vi "XS Electrode Write To Buffer.vi"(0 "XS Electrode Grid Array":bool[][](array[boolean])=[[FALSE, FALSE, FALSE], [FALSE, FALSE, FALSE], [FALSE, FALSE, FALSE], [FALSE, FALSE, FALSE], [FALSE, FALSE, FALSE], [FALSE, FALSE, FALSE]], 1 "64-bitmask Input":u64 format="%064b") -> (5 "64-bitmask Output":u64 format="%064b")   [LabVIEW 2017]
doc: "This VI will map the XS electrode grid array to ON-OFF bits in tehe 64 bit data buffer.\n\nAn array constant in this VI maps the XS electrode grid positions to the required HV channels."
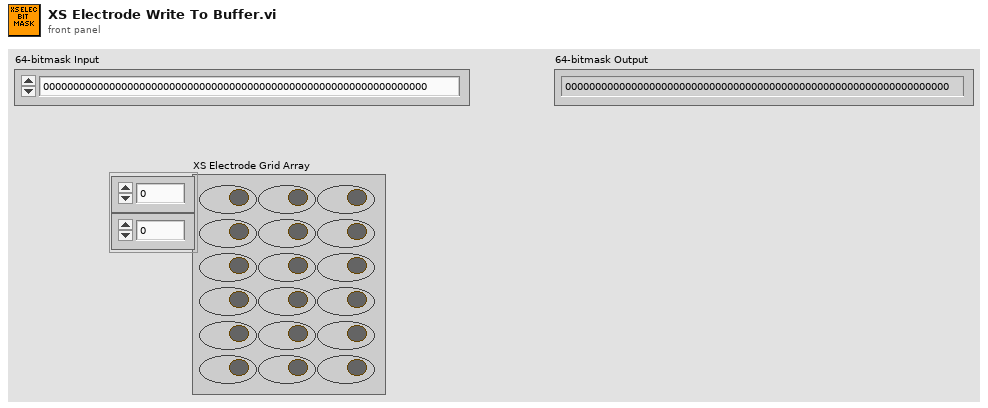
[diagram p1: front panel]
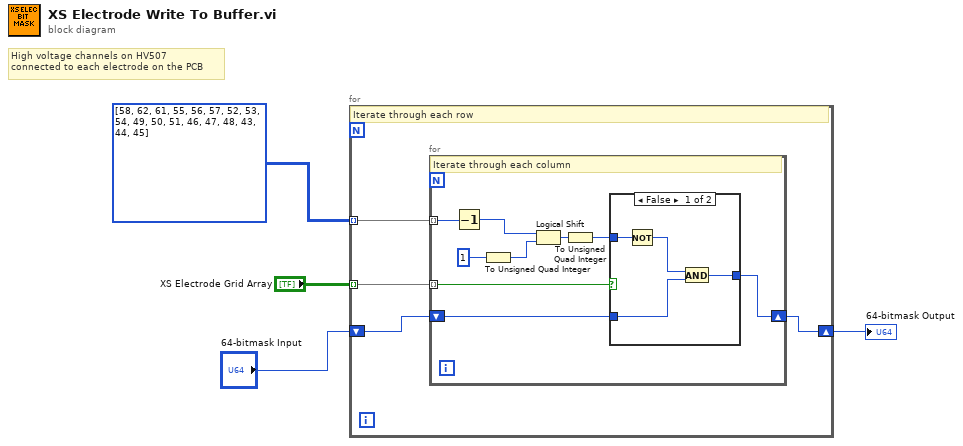
[diagram p0: block diagram]
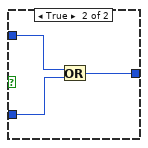
[diagram p2: hidden frame]
diagram:
  # "High voltage channels on HV507\nconnected to each electrode on the PCB"
  n1 = for {
    shift-right: [w7] -> w4
    shift-left: "64-bitmask Input" -> [w8]
    tunnel: "XS Electrode Grid Array" -> [w6] mode=indexing
    tunnel: u8[][] [[58, 62, 61], [55, 56, 57], [52, 53, 54], [49, 50, 51], [46, 47, 48], [43, 44, 45]] -> [w5] mode=indexing
    # "Iterate through each row"
    n2 = for {
      shift-right: [w9] -> w7
      shift-left: w8 -> [w10]
      tunnel: w6 -> [w11] mode=indexing
      tunnel: w5 -> [w17] mode=indexing
      # "Iterate through each column"
      n3 = Decrement(x=w17) -> (x-1=w13:u8)
      n4 = To Unsigned Quad Integer(1:u64 1 ("number")) -> (0:w14:u64)
      n5 = Logical Shift(y=w13, x=w14) -> (x << y=w16:u64)
      n6 = To Unsigned Quad Integer(1:w16) -> (0:w15:u64)
      n7 = case shown="False" w11 {
        tunnel: [w18 w24] -> w9
        tunnel: w15 -> [w21 w23]
        tunnel: w10 -> [w19 w22]
        frame False {
          n8 = Not(x=w21) -> (.not. x?=w20:u64)
          n9 = And(x=w20, y=w19) -> (x .and. y?=w18:u64)
        }
        frame True {
          n10 = Or(x=w23, y=w22) -> (x .or. y?=w24:u64)
        }
      }
    }
  }
  "64-bitmask Output" <- w4
